vi "SubVi_Actualizar_Reporte.vi"(11 "Cluster In":T1) -> (3 "Cluster out":T1)   [LabVIEW 2017]
uses:
  Cluster_Inicial.ctl
  <vilib>/Modbus/master/Modbus Master.lvclass
  <vilib>/addons/_office/excel.llb/Excel Get Data (dbl).vi
  <vilib>/addons/_office/excel.llb/Excel Easy Table (str).vi
  <vilib>/Utility/NIReport.llb/NI_report.lvclass
  <vilib>/addons/_office/NI_ReportGenerationToolkit.lvlib
  <vilib>/Utility/NIReport.llb/Excel/NI_Excel.lvclass
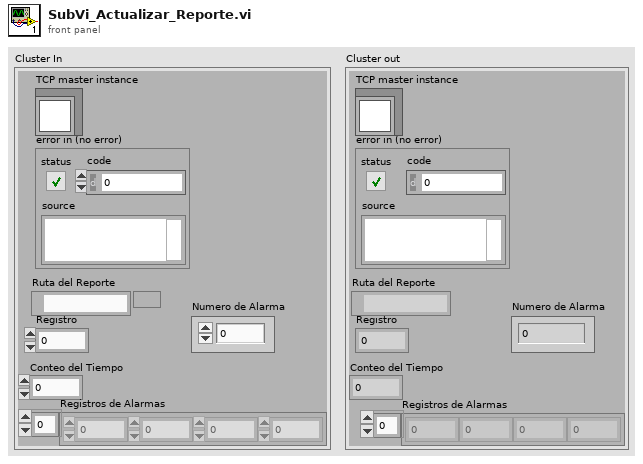
[diagram p1: front panel]
types:
  T1 = typedef "Cluster_Inicial.ctl" = cluster{"TCP master instance":refnum<class "Modbus Master.lvclass">, "error in (no error)":errorcluster, "Ruta del Reporte":path, "Registro":i32, "Conteo del Tiempo":i32, "Registros de Alarmas":i32[], "Numero de Alarma":u32}
  T2 = enum16{"maximized", "minimized", "normal", "no change"}
  T3 = enum16{"Standard Report", "HTML", "Word", "Excel"}
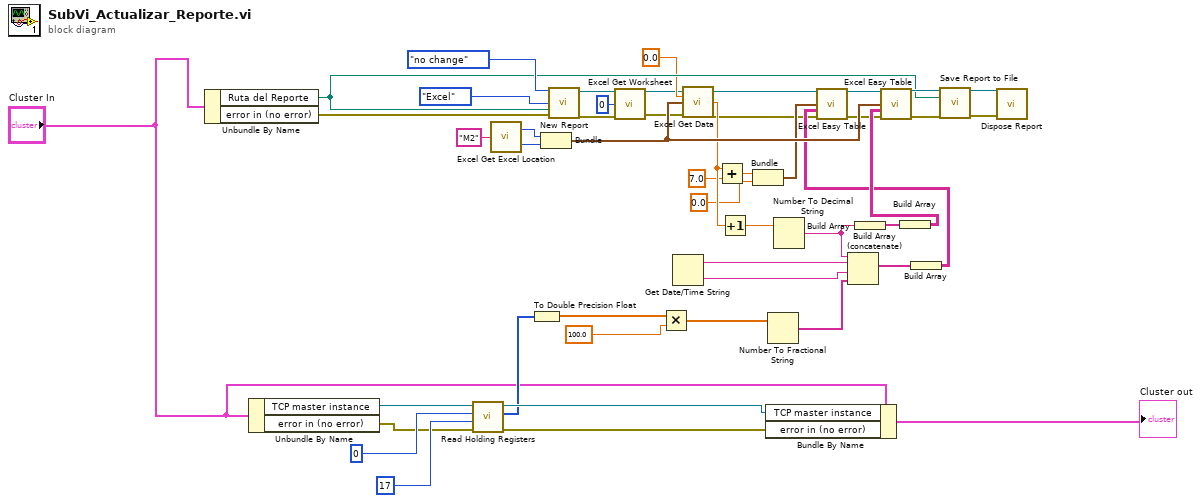
[diagram p0: block diagram]
diagram:
  n1 = Unbundle By Name("Cluster In") -> ("Ruta del Reporte"=w21:path, "error in (no error)"=w13:errorcluster)
  n2 = Unbundle By Name("Cluster In") -> ("TCP master instance"=w27:refnum<class "Modbus Master.lvclass">, "error in (no error)"=w28:errorcluster)
  n3 = call-dynamic "Read Holding Registers.vi"("error in (no error)"=w28, "number of holding registers"=u16 17, "starting address"=u16 0, "Modbus master in"=w27) -> ("error out"=w47:errorcluster, "register values"=w31:u16[], "Modbus master out"=w46:refnum<class "Modbus Master.lvclass">)  [unwired: 5 in]
  n4 = call <vilib>:"Excel Get Excel Location.vi"("cell's name"="M2") -> ("row"=w11:i32, "column"=w12:i32)
  n5 = To Double Precision Float(number=w31) -> (double precision float=w32:dbl[])
  n6 = Bundle("row"=w11, "column"=w12) -> (w41:cluster{"row":i32, "column":i32})  [unwired: 1 in]
  n7 = call <vilib>:"New Report.vi"("window state (normal)"=T2."no change", "report type"=T3."Excel", "template (empty)"=w21, "error in (no error)"=w13) -> ("report out"=w5:refnum<class "NI_report.lvclass">, "error out"=w6:errorcluster)  [unwired: 10 in]
  n8 = call <vilib>:"Excel Get Worksheet.vi"("report in"=w5, "worksheet index (0)"=0, "error in (no error)"=w6) -> ("report out"=w4:refnum<class "NI_report.lvclass">, "error out"=w3:errorcluster)  [unwired: 11 in]
  n9 = Multiply(x=w32, y=100.0) -> (x*y=w34:dbl[])
  n10 = Get Date/Time String() -> (date string=w35:string, time string=w36:string)  [unwired: 3 in]
  n11 = call-poly <vilib>:"Excel Get Data.vi"("report in"=w4, "data type"=0.0, "start (0, 0)"=w41, "error in (no error)"=w3) -> ("report out"=w1:refnum<class "NI_report.lvclass">, "data"=w22:dbl, "error out"=w2:errorcluster)  [unwired: 9 in]
  n12 = Add(x=w22, y=7.0) -> (x+y=w16:dbl)
  n13 = Increment(x=w22) -> (x+1=w23:dbl)
  n14 = Bundle(w16, 0.0) -> (w18:cluster{dbl, dbl})  [unwired: 1 in]
  n15 = Bundle By Name(cluster="Cluster In", "TCP master instance"=w46, "error in (no error)"=w47) -> (→"Cluster out":T1)
  n16 = Number To Fractional String(number=w34) -> (F-format string=w24:string[])  [unwired: 3 in]
  n17 = Number To Decimal String(number=w23) -> (decimal integer string=w42:string)  [unwired: 1 in]
  n18 = Build Array (concatenate)(w42, w35, w36, w24) -> (w25:string[])
  n19 = Build Array(w42) -> (w43:string[])
  n20 = Build Array(w43) -> (w44:string[][])
  n21 = Build Array(w25) -> (w26:string[][])
  n22 = call-poly <vilib>:"Excel Easy Table.vi"("report in"=w1, "start (0, 0)"=w18, "text data"=w26, "error in (no error)"=w2) -> ("report out"=w38:refnum<class "NI_report.lvclass">, "error out"=w39:errorcluster)  [unwired: 7 in, 3 out]
  n23 = call-poly <vilib>:"Excel Easy Table.vi"("report in"=w38, "start (0, 0)"=w41, "text data"=w44, "error in (no error)"=w39) -> ("report out"=w45:refnum<class "NI_report.lvclass">, "error out"=w40:errorcluster)  [unwired: 7 in, 3 out]
  n24 = call-dynamic "Save Report to File.vi"("report in"=w45, "report file path"=w21, "error in (no error)"=w40) -> ("report out"=w19:refnum<class "NI_report.lvclass">, "error out"=w20:errorcluster)  [unwired: 11 in]
  n25 = call-dynamic "Dispose Report.vi"("report in"=w19, "error in (no error)"=w20) -> ()  [unwired: 13 in, 1 out]
